vi "Write Timeout(s).vi"(8 "error in (no error)":errorcluster, 10 "Timeout(s)":i32, 11 "DAQ_Device in":refnum<class "DAQ_Device.lvclass">) -> (0 "error out":errorcluster, 3 "DAQ_Device out":refnum<class "DAQ_Device.lvclass">)   [LabVIEW 2023, in "DAQ_Device.lvclass"]
uses:
  DAQ_Device.lvclass
  DAQ_Device.lvclass/DAQ_Device.ctl
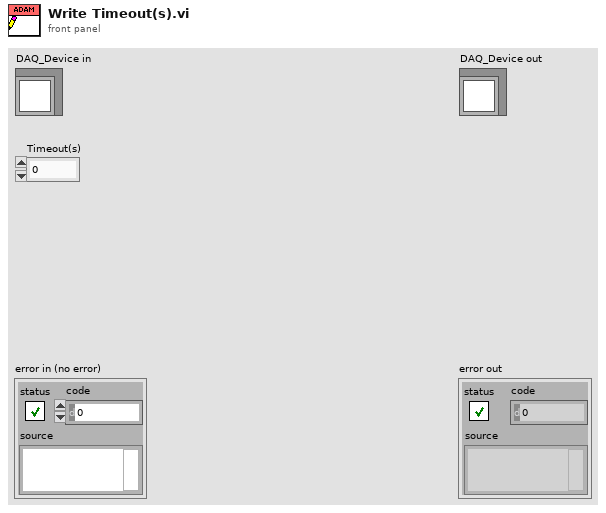
[diagram p1: front panel]
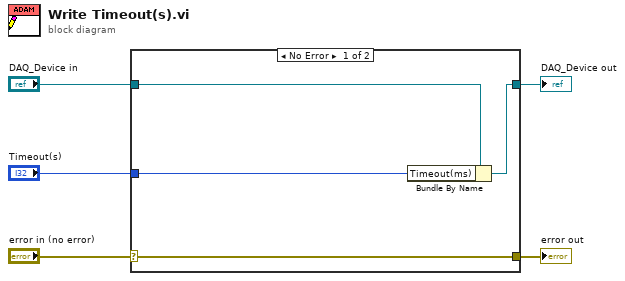
[diagram p0: block diagram]
diagram:
  n1 = case shown="No Error" "error in (no error)" {
    selector: "error in (no error)" -> [w9 w10]
    tunnel: [w9 w10] -> w4
    tunnel: [w7 w11] -> w2
    tunnel: "DAQ_Device in" -> [w8 w11]
    tunnel: "Timeout(s)" -> [w6 _]
    frame No Error {
      n2 = Bundle By Name(cluster=w8, "Timeout(ms)"=w6) -> (w7:refnum<class "DAQ_Device.lvclass">)
    }
    frame Error {
    }
  }
  "error out" <- w4
  "DAQ_Device out" <- w2
